vi "Read All Variables.vi"(8 "error in (no error)":errorcluster, 11 "Mapping params in":refnum<class "CV-Mapping.lvclass">) -> (0 "error out":errorcluster, 2 "Mapping vars.":T1, 3 "Mapping params out":refnum<class "CV-Mapping.lvclass">)   [LabVIEW 2013, in "CameraVision.lvlib" / "CV-Mapping.lvclass"]
uses:
  CV-Mapping.lvclass
  Mapping-variables.ctl
  UI/Module-states.ctl
  Mapping-characteristic.ctl
  CV-Mapping.lvclass/CV-Mapping.ctl
  UI/CV-UI.lvclass
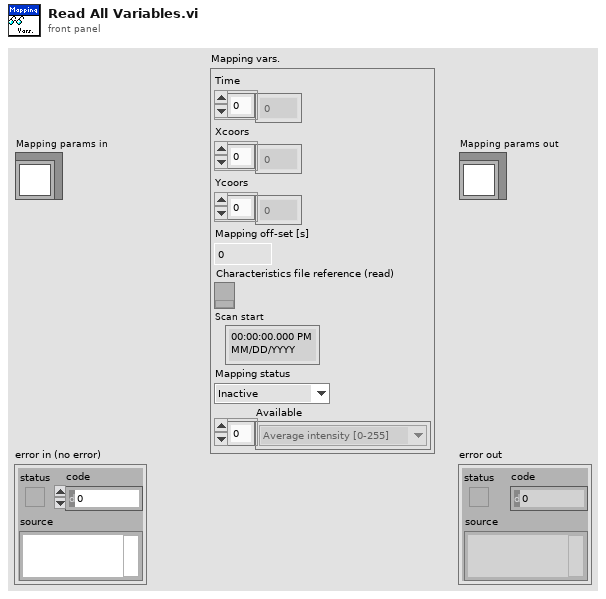
[diagram p1: front panel]
types:
  T1 = typedef "CameraVision.lvlib/CV-Mapping.lvclass/Mapping-variables.ctl" = cluster{"Time":sgl[], "Xcoors":sgl[], "Ycoors":sgl[], "Mapping off-set":dbl, "Characteristics file reference (read)":refnum<k34>, "Scan start":timestamp, "Mapping status":T2, "Available":T3[]}
  T2 = typedef "CameraVision.lvlib/CV-UI.lvclass/Module-states.ctl" = enum16{"Inactive", "Active", "Data-loss", "Error", "Simulation", "Synchronizing", "Initialized", "Released"}
  T3 = typedef "CameraVision.lvlib/CV-Mapping.lvclass/Mapping-characteristic.ctl" = enum16{"Average intensity [0-255]", "Peak intensity [0-255]", "Melt-pool size [mm²]", "Melt-pool aspect ratio []", "Melt-pool fragments []", "Average temperature [°C]", "Max. temperature [°C]", "Min. temperature [°C]", "Std. dev. temperature [°C]"}
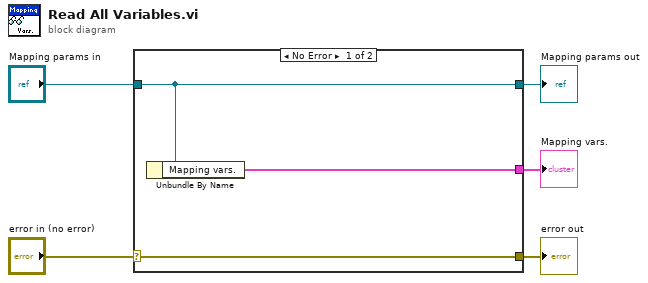
[diagram p0: block diagram]
diagram:
  n1 = case shown="No Error" "error in (no error)" {
    selector: "error in (no error)" -> [w8 w9]
    tunnel: [w8 w9] -> w4
    tunnel: [w7 w10] -> w2
    tunnel: "Mapping params in" -> [w7 w10]
    tunnel: [w6 _] -> w1
    frame No Error {
      n2 = Unbundle By Name(w7) -> ("Mapping vars."=w6:T1)
    }
    frame Error {
    }
  }
  "error out" <- w4
  "Mapping params out" <- w2
  "Mapping vars." <- w1
